vi "Periodic Tasks.vi"(8 "error in":errorcluster) -> ()   [LabVIEW 2018]
doc: "This VI runs in parallel to other tasks. It can contain as many user-defined periodic loops as you need. These can carry out PID or other sorts of timed response."
uses:
  <vilib>/Rock Robotics/WPI/Solenoid/WPI_SolenoidValue.ctl
  <vilib>/Rock Robotics/WPI/Utilities/WPI_GetSetVariantRefNum.vi
  <vilib>/Rock Robotics/Network Tables/NT Read String.vi
  Swerve/SwerveGlobals.vi
  <vilib>/Rock Robotics/WPI/Solenoid/WPI_SolenoidSetEnum.vi
  navx-mxp/labview/navX Library v2/navX Library v2.lvlib
panel:
  out "navX axes":T1
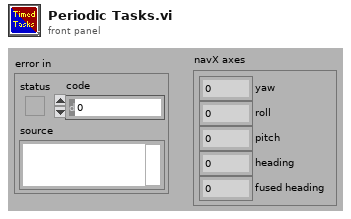
[diagram p1: front panel]
types:
  T1 = cluster{"yaw":dbl, "roll":dbl, "pitch":dbl, "heading":dbl, "fused heading":dbl}
  T2 = typedef "navX Library v2.lvlib/Z900_navX_DeviceTypeDef.ctl" = cluster{"Interface":cluster{"Protocol":T3, "Update Rate (4Hz-100Hz)":u8, "navX Open TypeDef":variant}, "Notify Packet":refnum<notifier>, "Loop VI Refnum":refnum<vi>, "Ready to Close Occurrence Refnum":refnum<k4>}
  T3 = typedef "navX Library v2.lvlib/Z900_navX_ProtocolTypeDef.ctl" = enum16{"SERIAL", "I2C", "SPI"}
  T4 = typedef "WPI_JoystickDevRef.ctl" = cluster{"Device":T5}
  T5 = typedef "WPI_JoystickDeviceEnum.ctl" = enum16{"USB 0", "USB 1", "USB 2", "USB 3", "USB 4", "USB 5"}
  T6 = typedef "WPI_AnalogChannelDevRef.ctl" = cluster{"DevStatus":errorcluster, "Analog Channel":T7}
  T7 = typedef "FPGA_AIChannel.ctl" = enum8{"AI 0", "AI 1", "AI 2", "AI 3", "AI MXP 0", "AI MXP 1", "AI MXP 2", "AI MXP 3", "Invalid"}
  T8 = typedef "WPI_MotorControlDeviceRef.ctl" = cluster{"DeviceStatus":errorcluster, "Type":T9, "PWM":cluster{"PWM Channel":T10, "DeadBand":T11}, "CAN":cluster{"Device Number":u8, "SetOutput VI Ref":variant, "GetOutput VI Ref":variant, "Enable VI Ref":variant, "Disable VI Ref":variant, "Data":variant}, "Invert":bool, "DIO PWM":cluster{"PWM \"Enable\" Channel":T10, "DIOChannel":T12, "PWM Rate":dbl}}
  T9 = typedef "WPI_MotorControlType.ctl" = enum16{"PWM", "CAN", "DIO PWM"}
  T10 = typedef "FPGA_DIOPWMChannel.ctl" = enum8{"PWM 0", "PWM 1", "PWM 2", "PWM 3", "PWM 4", "PWM 5", "PWM 6", "PWM 7", "PWM 8", "PWM 9", "PWM MXP 0", "PWM MXP 1", "PWM MXP 2", "PWM MXP 3", "PWM MXP 4", "PWM MXP 5", "PWM MXP 6", "PWM MXP 7", "PWM MXP 8", "PWM MXP 9", "Invalid"}
  T11 = typedef "WPI_PWMDeadband.ctl" = cluster{"Name":string, "maxPositivePwm":i32, "minPositivePwm":i32, "centerPwm":i32, "maxNegativePwm":i32, "minNegativePwm":i32, "angularRange":u16}
  T12 = typedef "FPGA_DIOChannel.ctl" = enum8{"DIO 0", "DIO 1", "DIO 2", "DIO 3", "DIO 4", "DIO 5", "DIO 6", "DIO 7", "DIO 8", "DIO 9", "DIO MXP 0", "DIO MXP 1", "DIO MXP 2", "DIO MXP 3", "DIO MXP 4", "DIO MXP 5", "DIO MXP 6", "DIO MXP 7", "DIO MXP 8", "DIO MXP 9", "DIO MXP 10", "DIO MXP 11", "DIO MXP 12", "DIO MXP 13", "DIO MXP 14", "DIO MXP 15", "SPI Port CS1", "SPI Port CS2", "SPI Port CS3", "SPI Port MISO", "SPI Port MOSI", "Invalid"}
  T13 = typedef "WPI_EncoderDevRef.ctl" = cluster{"DevStatus":errorcluster, "EncoderIndex":T14, "CounterIndex":T15, "DistancePerCount":dbl, "Decoding Type":T16}
  T14 = typedef "FPGA_EncoderIdx.ctl" = enum8{"Enc 0", "Enc 1", "Enc 2", "Enc 3", "Enc 4", "Enc 5", "Enc 6", "Enc 7", "Invalid"}
  T15 = typedef "FPGA_CounterCtrSystemIndex.ctl" = enum8{"Ctr 0", "Ctr 1", "Ctr 2", "Ctr 3", "Ctr 4", "Ctr 5", "Ctr 6", "Ctr 7", "Invalid"}
  T16 = typedef "WPI_EncoderType.ctl" = enum16{"1x", "2x", "4x"}
  T17 = typedef "WPI_SolenoidDevRef.ctl" = cluster{"DevStatus":errorcluster, "Pneumatics Control Module":u8, "Forward Solenoid Channel":T18, "Reverse Solenoid Channel":T18}
  T18 = typedef "WPI_SolenoidChannel.ctl" = enum8{"Solenoid 0", "Solenoid 1", "Solenoid 2", "Solenoid 3", "Solenoid 4", "Solenoid 5", "Solenoid 6", "Solenoid 7", "Invalid"}
  T19 = typedef "WPI_SolenoidValue.ctl" = enum16{"Off", "On", "Forward", "Reverse"}
  T20 = cluster{"Velocity X":dbl, "Velocity Y":dbl, "Velocity Z":dbl, "Displacement X":dbl, "Displacement Y":dbl, "Displacement Z":dbl}
  T21 = cluster{"Yaw":dbl, "Roll":dbl, "Pitch":dbl, "Heading":dbl, "Fused Heading":dbl}
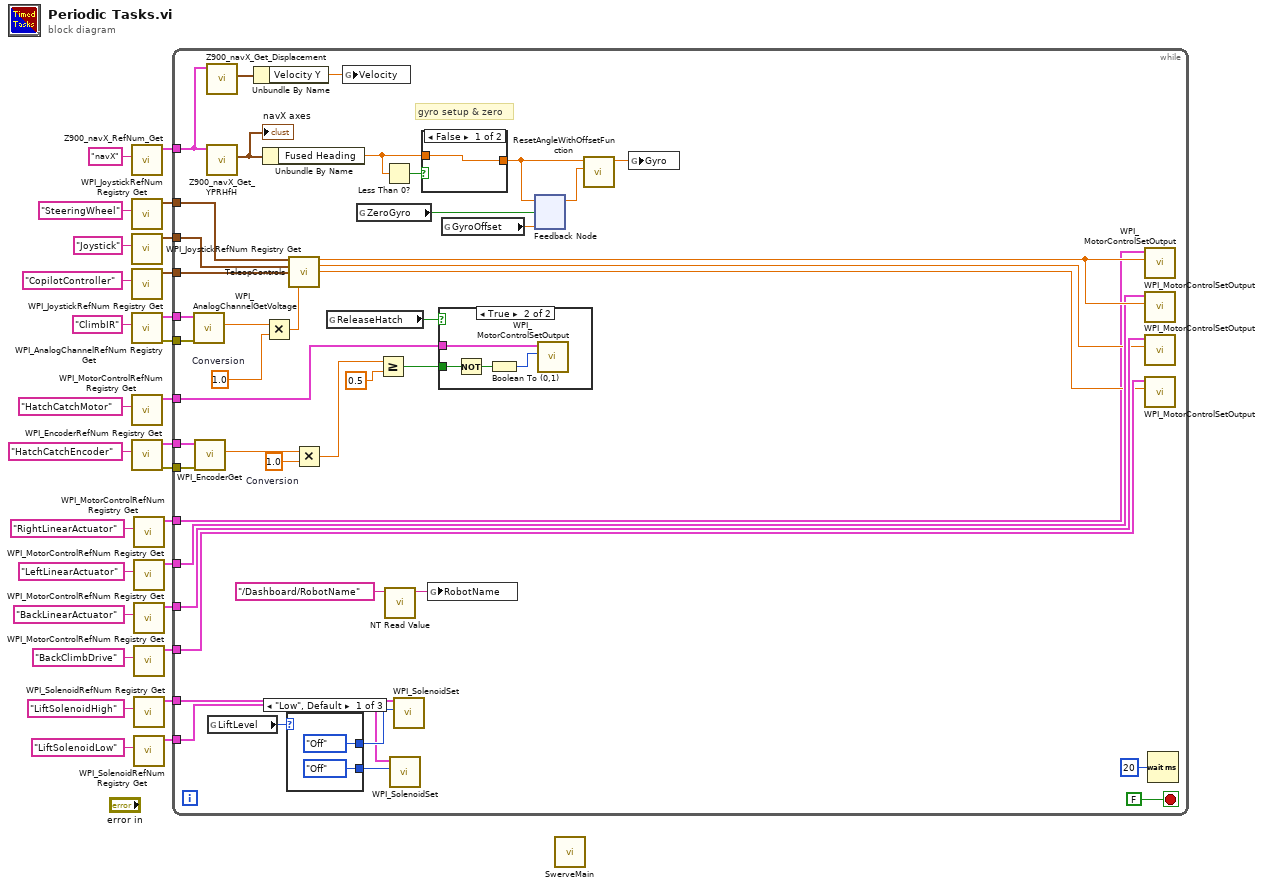
[diagram p0: block diagram]
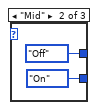
[diagram p2: hidden frame]
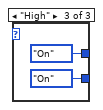
[diagram p3: hidden frame]
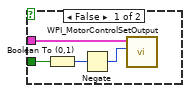
[diagram p4: hidden frame]
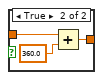
[diagram p5: hidden frame]
diagram:
  n1 = call "Z900_navX_RefNum_Get.vi"("refnum name"="navX") -> ("navX Device"=w27:T2)  [unwired: 9 in, 1 out]
  n2 = call <vilib>:"WPI_JoystickRefNum Registry Get.vi"("refnum name"="SteeringWheel") -> ("JoystickDevRef"=w23:T4)  [unwired: 1 in, 9 out]
  n3 = call <vilib>:"WPI_JoystickRefNum Registry Get.vi"("refnum name"="Joystick") -> ("JoystickDevRef"=w22:T4)  [unwired: 1 in, 9 out]
  n4 = call <vilib>:"WPI_JoystickRefNum Registry Get.vi"("refnum name"="CopilotController") -> ("JoystickDevRef"=w21:T4)  [unwired: 1 in, 9 out]
  n5 = call <vilib>:"WPI_AnalogChannelRefNum Registry Get.vi"("refnum name"="ClimbIR") -> ("error out"=w18:errorcluster, "AIDeviceRef"=w19:T6)  [unwired: 9 in]
  n6 = call <vilib>:"WPI_MotorControlRefNum Registry Get.vi"("refnum name"="HatchCatchMotor") -> ("MotorControlDevRef"=w13:T8)  [unwired: 9 in, 1 out]
  n7 = call <vilib>:"WPI_EncoderRefNum Registry Get.vi"("refnum name"="HatchCatchEncoder") -> ("error out"=w1:errorcluster, "EncoderDevRef"=w2:T13)  [unwired: 9 in]
  n8 = call <vilib>:"WPI_MotorControlRefNum Registry Get.vi"("refnum name"="RightLinearActuator") -> ("MotorControlDevRef"=w17:T8)  [unwired: 9 in, 1 out]
  n9 = call <vilib>:"WPI_MotorControlRefNum Registry Get.vi"("refnum name"="LeftLinearActuator") -> ("MotorControlDevRef"=w16:T8)  [unwired: 9 in, 1 out]
  n10 = call <vilib>:"WPI_MotorControlRefNum Registry Get.vi"("refnum name"="BackLinearActuator") -> ("MotorControlDevRef"=w15:T8)  [unwired: 9 in, 1 out]
  n11 = call <vilib>:"WPI_MotorControlRefNum Registry Get.vi"("refnum name"="BackClimbDrive") -> ("MotorControlDevRef"=w14:T8)  [unwired: 9 in, 1 out]
  n12 = call <vilib>:"WPI_SolenoidRefNum Registry Get.vi"("refnum name"="LiftSolenoidHigh") -> ("SolenoidDevRef"=w8:T17)  [unwired: 9 in, 1 out]
  n13 = call <vilib>:"WPI_SolenoidRefNum Registry Get.vi"("refnum name"="LiftSolenoidLow") -> ("SolenoidDevRef"=w7:T17)  [unwired: 9 in, 1 out]
  n14 = while {
    tunnel: w27 -> [w61]
    tunnel: w23 -> [w37]
    tunnel: w22 -> [w38]
    tunnel: w21 -> [w39]
    tunnel: w19 -> [w57]
    tunnel: w18 -> [w55]
    tunnel: w17 -> [w40]
    tunnel: w16 -> [w51]
    tunnel: w15 -> [w50]
    tunnel: w14 -> [w49]
    tunnel: w13 -> [w48]
    tunnel: w8 -> [w41]
    tunnel: w7 -> [w42]
    tunnel: w2 -> [w35]
    tunnel: w1 -> [w34]
    stop <- FALSE stop-if-true
    w32 = 1.0  # Conversion
    w54 = 1.0  # Conversion
    # "gyro setup & zero"
    n15 = call <vilib>:"WPI_AnalogChannelGetVoltage.vi"("error in (no error)"=w55, "AIDeviceRef"=w57) -> ("Voltage"=w56:dbl)  [unwired: 7 in, 2 out]
    n16 = call <vilib>:"WPI_EncoderGet.vi"("error in (no error)"=w34, "EncoderDevRef"=w35) -> ("Distance"=w33:dbl)  [unwired: 4 in, 5 out]
    n17 = call "Z900_navX_Get_Displacement.vi"("navX Device"=w61) -> ("Displacement"=w62:T20)  [unwired: 7 in, 3 out]
    n18 = call "Z900_navX_Get_YPRHfH.vi"("navX Device"=w61) -> ("YRPHfH"=w65:T21)  [unwired: 7 in, 3 out]
    "navX axes" <- w65
    n19 = global read "SwerveGlobals.vi" "LiftLevel"() -> (w45:enum16{"Low", "Mid", "High"})
    n20 = Unbundle By Name(w62) -> ("Velocity Y"=w60:dbl)
    n21 = Unbundle By Name(w65) -> ("Fused Heading"=w66:dbl)
    n22 = Multiply(x=w56, y=w54) -> (x*y=w36:dbl)
    n23 = case shown="\"Low\", Default" w45 {
      tunnel: [WPI_SolenoidValue."Off" ("Value") WPI_SolenoidValue."Off" ("Value") WPI_SolenoidValue."On" ("Value")] -> w44
      tunnel: [WPI_SolenoidValue."Off" ("Value") WPI_SolenoidValue."On" ("Value") WPI_SolenoidValue."On" ("Value")] -> w43
      frame "Low", Default {
      }
      frame "Mid" {
      }
      frame "High" {
      }
    }
    n24 = call "TeleopControls.vi"("SteeringWheelDefRef"=w37, "JoystickDevRef"=w38, "CopilotDevRef"=w39, "ClimbIRVal"=w36) -> ("ActuateFrontClimb"=w53:dbl, "ActuateBackClimb"=w46:dbl, "ClimbDrive"=w47:dbl)  [unwired: 9 in]
    n25 = Multiply(x=w33, y=w32) -> (x*y=w31:dbl)
    n26 = global read "SwerveGlobals.vi" "ReleaseHatch"() -> (w52:bool)
    n27 = global write "SwerveGlobals.vi" "Velocity"(w60) -> ()
    n28 = global read "SwerveGlobals.vi" "ZeroGyro"() -> (w63:bool)
    n29 = Greater Or Equal?(x=w31, y=0.5) -> (x >= y?=w29:bool)
    n30 = Less Than 0?(x=w66) -> (x < 0?=w70:bool)
    n31 = call-poly <vilib>:"NT Read Value.vi"("Name"="/Dashboard/RobotName") -> ("String"=w59:string)  [unwired: 9 in, 1 out]
    n32 = call-poly <vilib>:"WPI_SolenoidSet.vi"("Value"=w43, "SolenoidDevRef"=w42) -> ()  [unwired: 8 in, 2 out]
    n33 = call-poly <vilib>:"WPI_SolenoidSet.vi"("Value"=w44, "SolenoidDevRef"=w41) -> ()  [unwired: 8 in, 2 out]
    n34 = case shown="False" w70 {
      tunnel: w66 -> [w87 w90]
      tunnel: [w87 w88] -> w67
      frame False {
      }
      frame True {
        n35 = Add(x=w90, y=360.0) -> (x+y=w88:dbl)
      }
    }
    n36 = global write "SwerveGlobals.vi" "RobotName"(w59) -> ()
    n37 = case shown="True" w52 {
      tunnel: w48 -> [w82 w84]
      tunnel: w29 -> [w79 w83]
      frame False {
        n38 = Boolean To (0,1)(Boolean=w79) -> (0, 1=w81:i16)
        n39 = Negate(x=w81) -> (-x=w80:i16)
        n40 = call <vilib>:"WPI_MotorControlSetOutput.vi"("Output"=w80, "MotorControlDevRef"=w82) -> ()  [unwired: 7 in, 3 out]
      }
      frame True {
        n41 = Not(x=w83) -> (.not. x?=w86:bool)
        n42 = Boolean To (0,1)(Boolean=w86) -> (0, 1=w85:i16)
        n43 = call <vilib>:"WPI_MotorControlSetOutput.vi"("Output"=w85, "MotorControlDevRef"=w84) -> ()  [unwired: 7 in, 3 out]
      }
    }
    n44 = global read "SwerveGlobals.vi" "GyroOffset"() -> (w69:dbl)
    n45 = feedback-in #1(w67, w63) -> ()
    n46 = feedback #1(w69) -> (w68:dbl)
    n47 = call "ResetAngleWithOffsetFunction.vi"("Offset"=w68, "AngleInput"=w67) -> ("AngleOutput"=w64:dbl)  [unwired: 9 in]
    n48 = global write "SwerveGlobals.vi" "Gyro"(w64) -> ()
    n49 = call <vilib>:"WPI_MotorControlSetOutput.vi"("Output"=w53, "MotorControlDevRef"=w40) -> ()  [unwired: 7 in, 3 out]
    n50 = call <vilib>:"WPI_MotorControlSetOutput.vi"("Output"=w53, "MotorControlDevRef"=w51) -> ()  [unwired: 7 in, 3 out]
    n51 = call <vilib>:"WPI_MotorControlSetOutput.vi"("Output"=w46, "MotorControlDevRef"=w50) -> ()  [unwired: 7 in, 3 out]
    n52 = call <vilib>:"WPI_MotorControlSetOutput.vi"("Output"=w47, "MotorControlDevRef"=w49) -> ()  [unwired: 7 in, 3 out]
    n53 = Wait (ms)(milliseconds to wait=u32 20) -> ()  [unwired: 1 out]
  }
  n54 = call "SwerveMain.vi"() -> ()  [unwired: 12 in]
